vi "x502_gen_signal.vi"(1 "Channel 2 Signal Params":T1(array[cluster]), 2 "Channel 1 Signal Params":T1(array[cluster]), 3 "Gen Freq":dbl) -> (0 "Generated Points":dbl[][](array[numeric]))   [LabVIEW 2010]
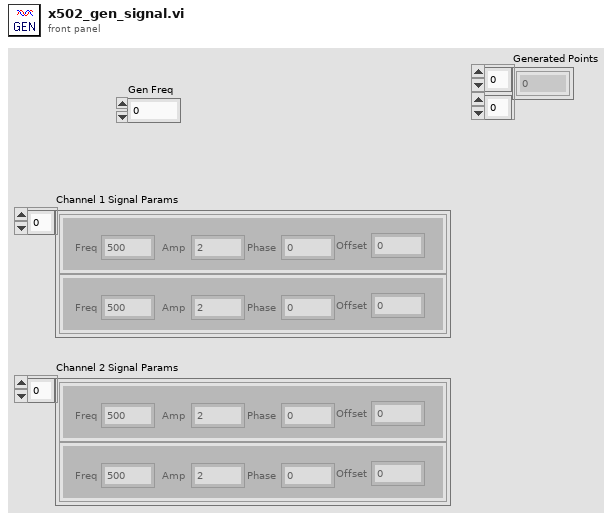
[diagram p1: front panel]
types:
  T1 = cluster{"Freq":dbl, "Amp":dbl, "Phase":dbl, "Offset":dbl}[]
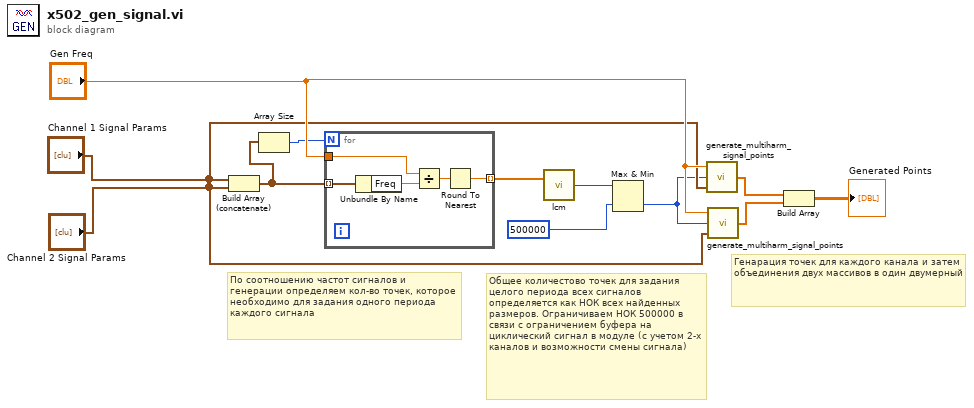
[diagram p0: block diagram]
diagram:
  # "Генарация точек для каждого канала и затем объединения двух массивов в один двумерный"
  # "Общее количестово точек для задания целого периода всех сигналов определяется как НОК всех найденных размеров. Ограничиваем НОК 500000 в связи с ограничением буфера на циклический сигнал в модуле (с учетом 2-х каналов и возможности смены сигнала)"
  # "По соотношению частот сигналов и генерации определяем кол-во точек, которое необходимо для задания одного периода каждого сигнала"
  n1 = Build Array (concatenate)("Channel 1 Signal Params", "Channel 2 Signal Params") -> (w6:T1)
  n2 = Array Size(array=w6) -> (size(s)=w5:i32)
  n3 = for {
    N: w5 -> [_]
    tunnel: w6 -> [w17] mode=indexing
    tunnel: "Gen Freq" -> [w15]
    tunnel: [w13] -> w4 mode=indexing
    n4 = Unbundle By Name(w17) -> ("Freq"=w16:dbl)
    n5 = Divide(x=w15, y=w16) -> (x/y=w14:dbl)
    n6 = Round To Nearest(number=w14) -> (nearest integer value=w13:dbl)
  }
  n7 = call "lcm.vi"("Values"=w4) -> ("LCM"=w3:i32)  [unwired: 1 in]
  n8 = Max & Min(x=w3, y=500000) -> (min(x,y)=w1:i32)  [unwired: 1 out]
  n9 = call "generate_multiharm_signal_points.vi"("Harmonics"="Channel 1 Signal Params", "Points Count"=w1, "Fout"="Gen Freq") -> ("Signal Points"=w9:dbl[])
  n10 = call "generate_multiharm_signal_points.vi"("Harmonics"="Channel 2 Signal Params", "Points Count"=w1, "Fout"="Gen Freq") -> ("Signal Points"=w8:dbl[])
  n11 = Build Array(w9, w8) -> (→"Generated Points":dbl[][])
